vi "BuildMessagesFromPicture.vi"(8 "error in (no error)":errorcluster, 11 "2D Picture":picture) -> (0 "error out":errorcluster, 3 "Messages":string[](array[string]))   [LabVIEW 2020, in "CTI-Peripheral.lvlib" / "64x128 I2C OLED SSD1315.lvclass"]
uses:
  64x128 I2C OLED SSD1315.lvclass
  64x128 I2C OLED SSD1315.lvclass/64x128 I2C OLED SSD1315.ctl
panel:
  # "Input"
  # "Output"
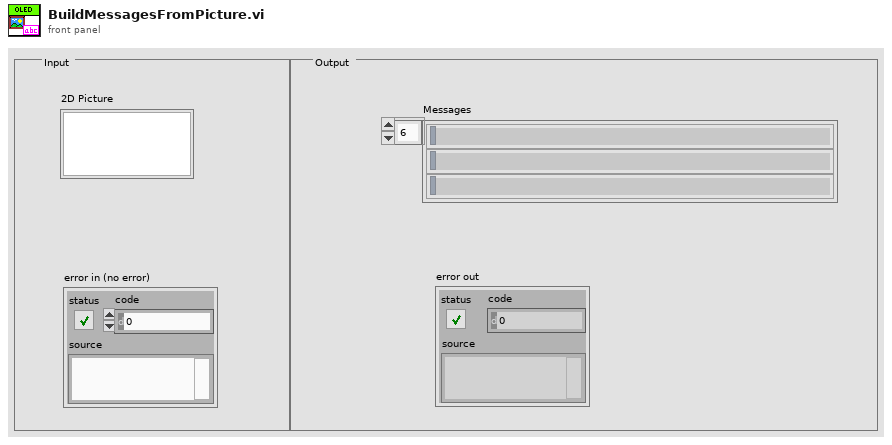
[diagram p1: front panel]
types:
  T1 = cluster{"left":i16, "top":i16, "right":i16, "bottom":i16}
  T2 = typedef "imagedata.ctl" = cluster{"image type":i32, "image depth":i32, "image":u8[], "mask":u8[], "colors":u32[], "Rectangle":cluster{"left":i16, "top":i16, "right":i16, "bottom":i16}}
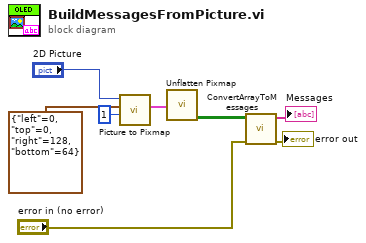
[diagram p0: block diagram]
diagram:
  n1 = call <vilib>:"Picture to Pixmap.vi"("depth"=1, "rect"=T1 {"left"=0, "top"=0, "right"=128, "bottom"=64}, "picture"="2D Picture") -> ("image data"=w7:T2)  [unwired: 7 in, 1 out]
  n2 = call <vilib>:"Unflatten Pixmap.vi"("image data"=w7) -> ("1-bit pixmap"=w4:bool[][])  [unwired: 4 in, 6 out]
  n3 = call "ConvertArrayToMessages.vi"("error in (no error)"="error in (no error)", "Array"=w4) -> ("error out"=→"error out":errorcluster, "Messages"=→"Messages":string[])  [unwired: 8 in]
